vi "4Pi Dual DM - Threshold 2D Array.vi"(0 "2D Array IN":dbl[][](array[numeric]), 7 "Upper Limit (Inclusive)":dbl, 11 "Lower Limit (Inclusive)":dbl) -> (8 "Threshold Array Out":dbl[](array[numeric]))   [LabVIEW 2021]
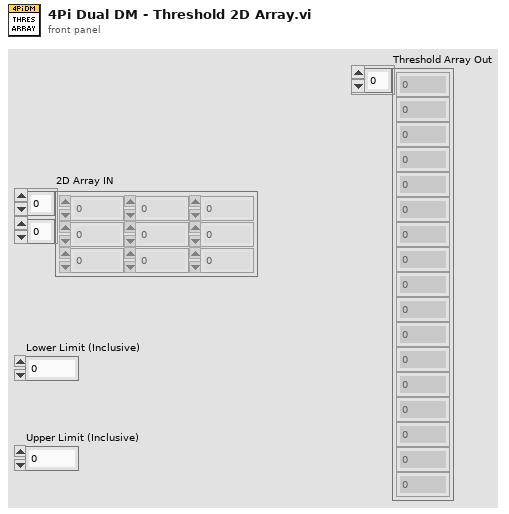
[diagram p1: front panel]
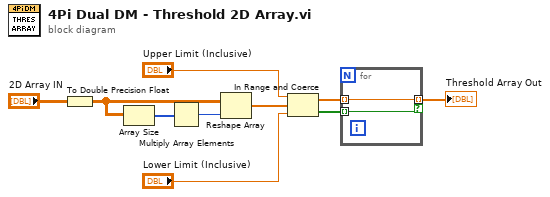
[diagram p0: block diagram]
diagram:
  n1 = To Double Precision Float(number="2D Array IN") -> (double precision float=w10:dbl[][])
  n2 = Array Size(array=w10) -> (size(s)=w8:i32[])
  n3 = Multiply Array Elements(1:w8) -> (0:w9:i32)
  n4 = Reshape Array(w10, w9) -> (w4:dbl[])
  n5 = In Range and Coerce(upper limit="Upper Limit (Inclusive)", x=w4, lower limit="Lower Limit (Inclusive)") -> (coerced(x)=w3:dbl[], In Range?=w2:bool[])
  n6 = for {
    tunnel: w3 -> [w12] mode=indexing
    tunnel: w2 -> [w11] mode=indexing
    tunnel: [w12] -> w1 mode=indexing if=w11
  }
  "Threshold Array Out" <- w1
